vi "DatabaseHand_Dequeue.vi"(4 "non-destructive queue":bool, 6 "queue?":bool, 7 "unit in":string, 9 "value in":string, 10 "name":string) -> (2 "value out":string, 5 "unit out":string)   [LabVIEW 2016]
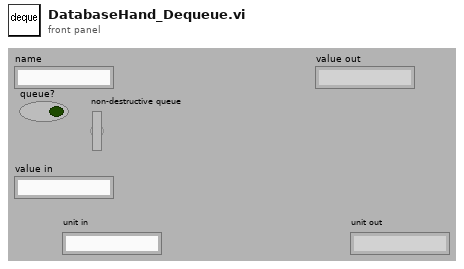
[diagram p1: front panel]
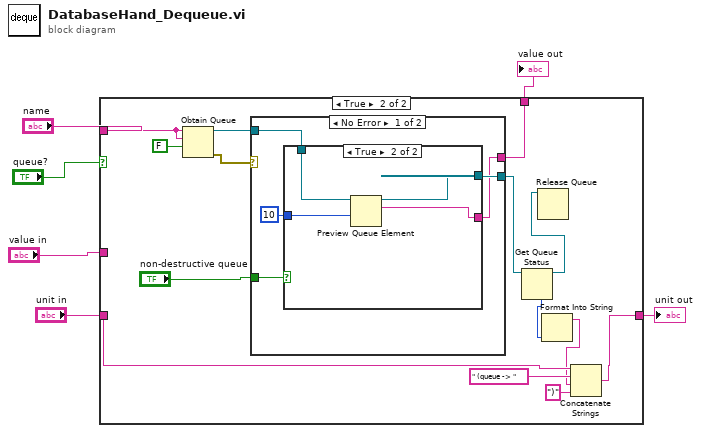
[diagram p0: block diagram]
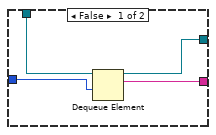
[diagram p3: hidden frame]
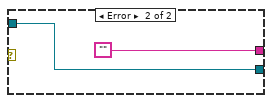
[diagram p4: hidden frame]
diagram:
  n1 = case shown="True" "queue?" {
    tunnel: [w8 w17] -> w5
    tunnel: "name" -> [_ w22]
    tunnel: "value in" -> [w8 _]
    tunnel: [w7 w14] -> w2
    tunnel: "unit in" -> [w7 w16]
    frame False {
    }
    frame True {
      n2 = Obtain Queue(name (unnamed)=w22, element data type=w22, create if not found? (T)=FALSE) -> (queue out=w18:refnum<queue>, error out=w20:errorcluster)  [unwired: 2 in, 1 out]
      n3 = case shown="No Error" w20 {
        tunnel: "non-destructive queue" -> [w27 _]
        tunnel: [w26 w37] -> w13
        tunnel: w18 -> [w25 w37]
        tunnel: [w24 ""] -> w17
        frame No Error {
          n4 = case shown="True" w27 {
            tunnel: [w30 w33] -> w26
            tunnel: w25 -> [w31 w35]
            tunnel: [w29 w34] -> w24
            tunnel: 10 ("timeout in ms (-1)") -> [w28 w32]
            frame False {
              n5 = Dequeue Element(queue=w31, timeout in ms (-1)=w28) -> (queue out=w30:refnum<queue>, element=w29:string)  [unwired: 1 in, 2 out]
            }
            frame True {
              n6 = Preview Queue Element(queue=w35, timeout in ms (-1)=w32) -> (queue out=w33:refnum<queue>, element=w34:string)  [unwired: 1 in, 2 out]
            }
          }
        }
        frame Error {
        }
      }
      n7 = Get Queue Status(queue=w13) -> (queue out=w12:refnum<queue>, # elements in queue=w11:i32)  [unwired: 1 in, 7 out]
      n8 = Release Queue(queue=w12) -> ()  [unwired: 1 in, 4 out]
      n9 = Format Into String(w11) -> (resulting string=w10:string)  [unwired: 3 in, 1 out]
      n10 = Concatenate Strings(w16, " (queue -> " ("string"), w10, ")" ("string")) -> (w14:string)
    }
  }
  "value out" <- w5
  "unit out" <- w2
